vi "Renishaw-XL80_GetSerialNumber.vi"(8 "error in (no error)":errorcluster, 11 "Renishaw-XL80 in":refnum<class "Renishaw-XL80.lvclass">) -> (0 "error out":errorcluster, 2 "DX10SerialNumber":string, 3 "Renishaw-XL80 out":refnum<class "Renishaw-XL80.lvclass">)   [LabVIEW 2024, in "Renishaw-XL80.lvclass"]
doc: "This read only property returns the serial number of the DX10.\n\nDefinition\nHRESULTget_DX10SerialNumber( [out, retval] BSTR* pVal);\nParameters\npVal\nA variable that will be set to the serial number of the DX10. \nComments\nThis property will return an empty string if the client has not previously connected to a DX10 by calling Connect.\n\nThe property will normally return an HRESULT of S_OK. However, it will return E_POINTER if the client supplies a null pointer for pVal, and in extremely low memory conditions it will return E_NOMEMORY.\n\nSee Also"
uses:
  Renishaw-XL80.lvclass
  Renishaw-XL80.lvclass/Renishaw-XL80.ctl
  D:/A.C.M/Example CSharp_64/bin/Debug/Interop.DX10SDKADAPTORLib.dll
  Example CSharp_64/bin/Debug/Interop.DX10SDKADAPTORLib.dll
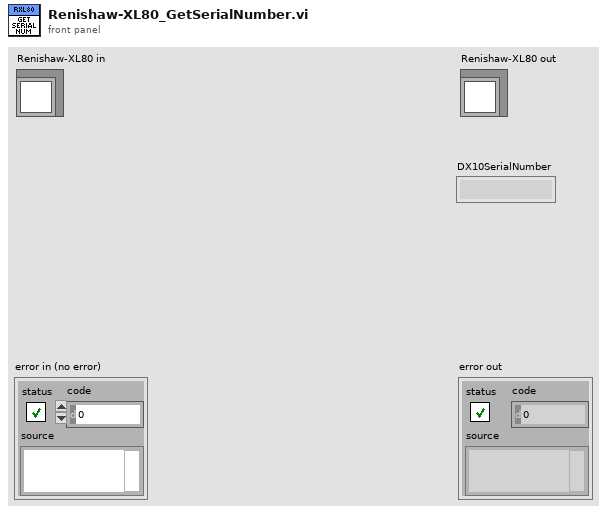
[diagram p1: front panel]
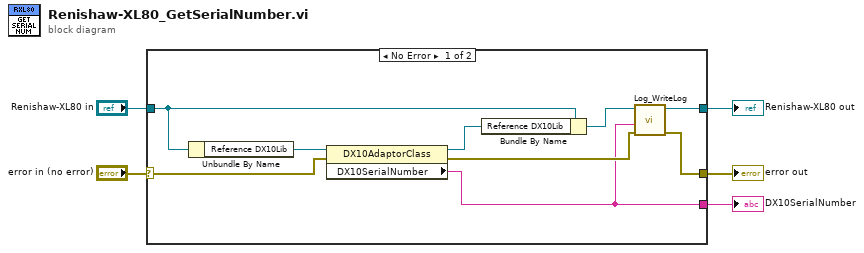
[diagram p0: block diagram]
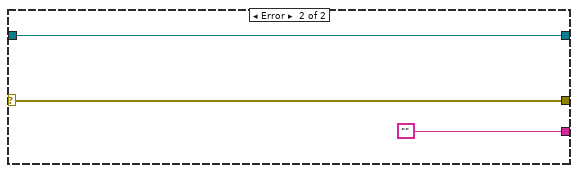
[diagram p2: hidden frame]
diagram:
  n1 = case shown="No Error" "error in (no error)" {
    selector: "error in (no error)" -> [w11 w17]
    tunnel: [w6 w17] -> w4
    tunnel: [w7 w16] -> w2
    tunnel: "Renishaw-XL80 in" -> [w13 w16]
    tunnel: [w9 ""] -> w1
    frame No Error {
      n2 = Unbundle By Name(w13) -> ("Reference DX10Lib"=w14:refnum<k24>)
      n3 = property class="DX10AdaptorClass"(reference=w14, error in=w11) -> (reference out=w12:refnum<k24>, error out=w10:errorcluster, "DX10SerialNumber"=w9:string)
      n4 = Bundle By Name(cluster=w13, "Reference DX10Lib"=w12) -> (w8:refnum<class "Renishaw-XL80.lvclass">)
      n5 = call-dynamic "Log_WriteLog.vi"("error in (no error)"=w10, "Response"=w9, "Log in"=w8) -> ("error out"=w6:errorcluster, "Log out"=w7:refnum<class "Renishaw-XL80.lvclass">)  [unwired: 7 in]
    }
    frame Error {
    }
  }
  "error out" <- w4
  "Renishaw-XL80 out" <- w2
  "DX10SerialNumber" <- w1
